vi "Flipper_Arb.vi"(0 "P1_Value":enum16{"Closed", "Open"}(ring), 1 "P1_Enable":bool, 2 "P3_Enable":bool, 5 "P2_Value":enum16{"Closed", "Open"}(ring), 7 "P3_Value":enum16{"Closed", "Open"}(ring), 9 "P4_Value":enum16{"Closed", "Open"}(ring), 12 "P2_Enable":bool, 13 "P4_Enable":bool) -> (4 "P_Out":enum16{"Closed", "Open"}(ring), 6 "Any True?":bool)   [LabVIEW 2015]
panel:
  # "P1 is highest priority\np5 is lowest"
  # "Josh Merkle 2/8/16"
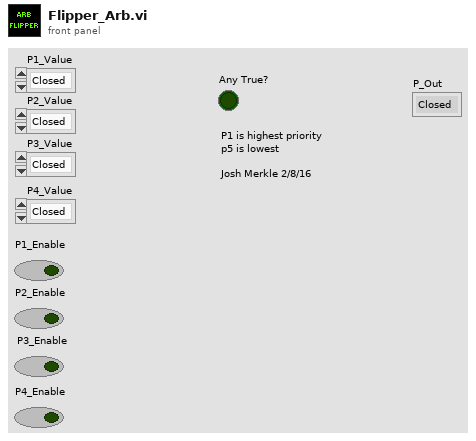
[diagram p1: front panel]
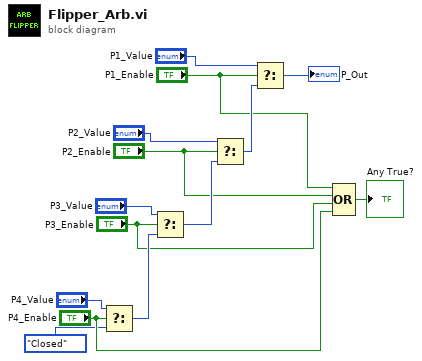
[diagram p0: block diagram]
diagram:
  n1 = Select(t="P4_Value", s="P4_Enable", f=enum16{"Closed", "Open"}."Closed" ("P3_Value 2")) -> (s? t:f=w14:enum16{"Closed", "Open"})
  n2 = Select(t="P3_Value", s="P3_Enable", f=w14) -> (s? t:f=w13:enum16{"Closed", "Open"})
  n3 = Select(t="P2_Value", s="P2_Enable", f=w13) -> (s? t:f=w12:enum16{"Closed", "Open"})
  n4 = Select(t="P1_Value", s="P1_Enable", f=w12) -> (s? t:f=→"P_Out":enum16{"Closed", "Open"})
  n5 = Compound Arithmetic op=OR("P1_Enable", "P2_Enable", "P3_Enable", "P4_Enable") -> (→"Any True?":bool)
